vi "Config SCPI Serial Port.vi"(8 "error in":errorcluster, 10 "Settings":T1={"Baud Rate"=enum."9600", "Timeout"=10000, "Stop Bits"=10, "Flow Control"=enum."None", "Parity"=0} {"Parity" items=["None", "Odd", "Even", "Mark", "Space"]; "Stop Bits" items=["1.0"=10, "1.5"=15, "2.0"=20]}, 11 "VISA Refnum in":refnum<visa-resource-name>) -> (0 "error out":errorcluster, 3 "VISA Refnum out":refnum<visa-resource-name>)   [LabVIEW 2021, in "Keysight U1282A.lvlib"]
uses:
  Keysight U1282A.lvlib
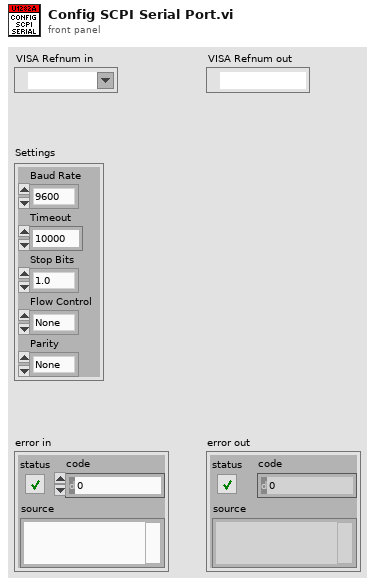
[diagram p1: front panel]
types:
  T1 = cluster{"Baud Rate":enum16{"1200", "2400", "4800", "9600", "19200", "38400", "57600", "115200"}, "Timeout":u32, "Stop Bits":u16, "Flow Control":enum16{"None", "XON / XOFF", "RTS / CTS", "DTR / DSR"}, "Parity":u16}
  T2 = enum16{"None", "XON / XOFF", "RTS / CTS", "DTR / DSR"}
  T3 = enum16{"1200", "2400", "4800", "9600", "19200", "38400", "57600", "115200"}
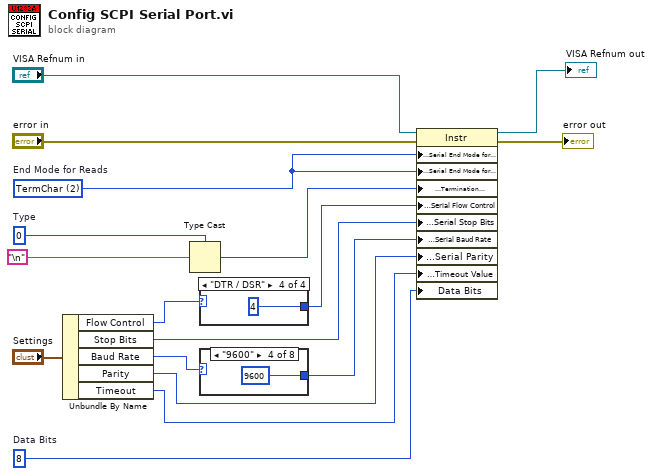
[diagram p0: block diagram]
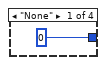
[diagram p2: hidden frame]
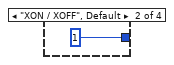
[diagram p3: hidden frame]
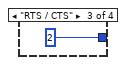
[diagram p4: hidden frame]
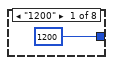
[diagram p5: hidden frame]
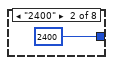
[diagram p6: hidden frame]
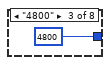
[diagram p7: hidden frame]
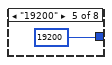
[diagram p8: hidden frame]
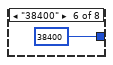
[diagram p9: hidden frame]
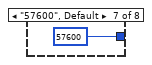
[diagram p10: hidden frame]
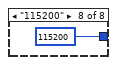
[diagram p11: hidden frame]
diagram:
  w8 = u16 2 items=["None", "Last Bit", "TermChar"]  # End Mode for Reads
  w1 = u16 8  # Data Bits
  w13 = u8 0  # Type
  n1 = Unbundle By Name("Settings") -> ("Flow Control"=w4:T2, "Stop Bits"=w5:u16, "Baud Rate"=w6:T3, "Parity"=w3:u16, "Timeout"=w2:u32)
  n2 = Type Cast(type=w13, x="\n" ("Line Feed Constant")) -> (*(type *) &x=w15:u8)
  n3 = case shown="\"DTR / DSR\"" w4 {
    tunnel: [u16 0 u16 1 u16 2 u16 4] -> w12
    frame "None" {
    }
    frame "XON / XOFF", Default {
    }
    frame "RTS / CTS" {
    }
    frame "DTR / DSR" {
    }
  }
  n4 = case shown="\"9600\"" w6 {
    tunnel: [u32 1200 u32 2400 u32 4800 u32 9600 u32 19200 u32 38400 u32 57600 u32 115200] -> w11
    frame "1200" {
    }
    frame "2400" {
    }
    frame "4800" {
    }
    frame "9600" {
    }
    frame "19200" {
    }
    frame "38400" {
    }
    frame "57600", Default {
    }
    frame "115200" {
    }
  }
  n5 = property on="Property Node" class="Instr"(reference="VISA Refnum in", error in="error in", "Serial Settings:Serial End Mode for Reads"=w8, "Serial Settings:Serial End Mode for Writes"=w8, "Message Based Settings:Termination Character"=w15, "Serial Settings:Serial Flow Control"=w12, "Serial Settings:Serial Stop Bits"=w5, "Serial Settings:Serial Baud Rate"=w11, "Serial Settings:Serial Parity"=w3, "General Settings:Timeout Value"=w2, "Data Bits"=w1) -> (reference out=→"VISA Refnum out":refnum<visa-resource-name>, error out=→"error out":errorcluster)
